vi "HTTPMethod_getHello.vi"(7 "LabVIEW Web Service Request":refnum<class "Web Request.lvclass">) -> (3 "Message":string="Hello World")   [LabVIEW 2020]
uses:
  <vilib>/wsapi/Web Request.lvclass
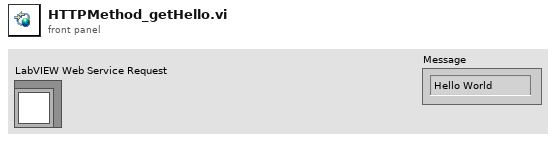
[diagram p1: front panel]
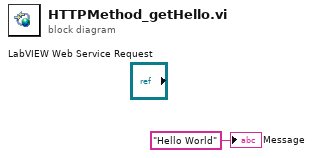
[diagram p0: block diagram]
diagram:
  "Message" <- "Hello World"
